vi "Tiles.vi"(4 "Properties":T1={"Colormap"={"Map"=enum."Automatic", "Value Min"=nan, "Value Max"=nan, "Scaling"=enum."Default", "Reverse"=FALSE}, "Line"={"Style"=enum."Automatic", "Color"=2147483647, "Width"=nan}, "Display"={"Alpha"=nan, "Z Order"=nan}} {"Line"."Color" items=["Automatic"=2147483647, "Black"=0, "White"=16777215, "Red"=16711680, "Green"=2263842, "Blue"=255, "Cyan"=65535, "Magenta"=16711935, "Yellow"=16776960]}, 7 "Z Data":dbl[][](array[numeric]), 8 "error in (no error)":errorcluster, 9 "Y Tile Boundaries":dbl[](array[numeric]), 10 "X Tile Boundaries":dbl[](array[numeric]), 11 "Plot ID":T9 format="%x") -> (0 "error out":errorcluster, 3 "Plot ID Out":T9 format="%x")   [LabVIEW 2013, in "Advanced Plotting Toolkit.lvlib"]
doc: "Display an array as a series of rectangular tiles, colored according to a colormap. Tile edge locations may optionally be specified."
uses:
  Advanced Plotting Toolkit.lvlib
  typedefs/PlotID.ctl
  TilesProperties.ctl
  properties/Colormap.ctl
  properties/Colormap_Map.ctl
  properties/Colormap_Scaling.ctl
  properties/Line.ctl
  properties/Line_Style.ctl
  typedefs/PlotColor.ctl
  properties/Display.ctl
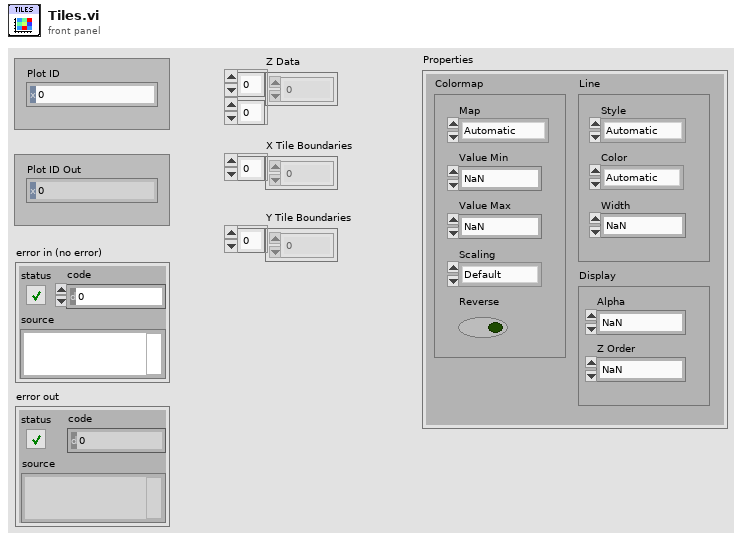
[diagram p1: front panel]
types:
  T1 = typedef "Advanced Plotting Toolkit.lvlib/TilesProperties.ctl" = cluster{"Colormap":T2, "Line":T5, "Display":T8}
  T2 = typedef "Advanced Plotting Toolkit.lvlib/Colormap.ctl" = cluster{"Map":T3, "Value Min":dbl, "Value Max":dbl, "Scaling":T4, "Reverse":bool}
  T3 = typedef "Advanced Plotting Toolkit.lvlib/Colormap_Map.ctl" = enum16{"Automatic", "Rainbow", "Hot and Cold", "White-Black", "White-Blue", "White-Green", "White-Red", "Fire", "Water", "Earth", "Air", "Pastel", "Banded", "Stepped"}
  T4 = typedef "Advanced Plotting Toolkit.lvlib/Colormap_Scaling.ctl" = enum16{"Default"}
  T5 = typedef "Advanced Plotting Toolkit.lvlib/Line.ctl" = cluster{"Style":T6, "Color":T7, "Width":sgl}
  T6 = typedef "Advanced Plotting Toolkit.lvlib/Line_Style.ctl" = enum16{"Automatic", "Solid", "Dashed", "Dotted", "Dash-dot", "Invisible"}
  T7 = typedef "Advanced Plotting Toolkit.lvlib/PlotColor.ctl" = u32
  T8 = typedef "Advanced Plotting Toolkit.lvlib/Display.ctl" = cluster{"Alpha":dbl, "Z Order":dbl}
  T9 = typedef "Advanced Plotting Toolkit.lvlib/PlotID.ctl" = i32
  T10 = typedef "Advanced Plotting Toolkit.lvlib/KeyValue.ctl" = cluster{"Key":string, "Value":string}
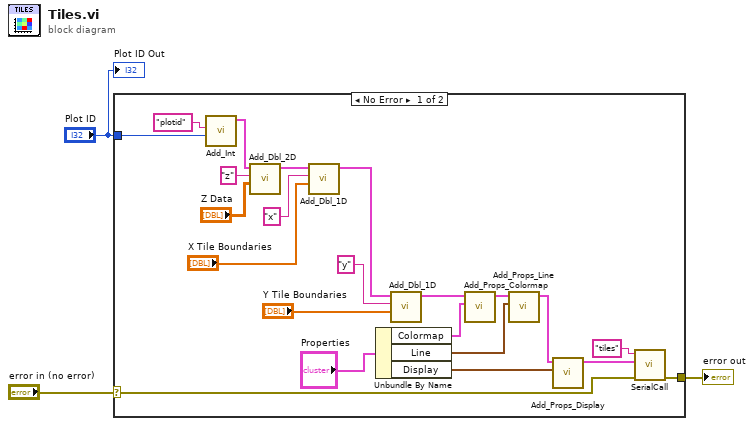
[diagram p0: block diagram]
diagram:
  n1 = case shown="No Error" "error in (no error)" {
    selector: "error in (no error)" -> [w15 w26]
    tunnel: "Plot ID" -> [w25 _]
    tunnel: [w14 w26] -> w1
    frame No Error {
      n2 = call "Add_Int.vi"("Value"=w25, "Key"="plotid") -> ("Keyword Array Out"=w20:T10[])  [unwired: 9 in]
      n3 = call "Add_Dbl_2D.vi"("Value"="Z Data", "Key"="z", "Keyword Array"=w20) -> ("Keyword Array Out"=w19:T10[])  [unwired: 8 in]
      n4 = call "Add_Dbl_1D.vi"("Value"="X Tile Boundaries", "Key"="x", "Keyword Array"=w19) -> ("Keyword Array Out"=w16:T10[])  [unwired: 8 in]
      n5 = Unbundle By Name("Properties") -> ("Colormap"=w4:T2, "Line"=w8:T5, "Display"=w7:T8)
      n6 = call "Add_Dbl_1D.vi"("Value"="Y Tile Boundaries", "Key"="y", "Keyword Array"=w16) -> ("Keyword Array Out"=w5:T10[])  [unwired: 8 in]
      n7 = call "Add_Props_Colormap.vi"("Colormap"=w4, "Keyword Array"=w5) -> ("Keyword Array Out"=w6:T10[])  [unwired: 9 in]
      n8 = call "Add_Props_Line.vi"("Line"=w8, "Keyword Array"=w6) -> ("Keyword Array Out"=w12:T10[])  [unwired: 9 in]
      n9 = call "Add_Props_Display.vi"("Display"=w7, "Keyword Array"=w12) -> ("Keyword Array Out"=w11:T10[])  [unwired: 9 in]
      n10 = call "SerialCall.vi"("error in (no error)"=w15, "data"=w11, "Resource"="tiles") -> ("error out"=w14:errorcluster)  [unwired: 7 in, 1 out]
    }
    frame Error {
    }
  }
  "error out" <- w1
  "Plot ID Out" <- "Plot ID"
